vi "Command (read & write) - PR.vi"(7 "timeout ms (100)":i32=100, 8 "error in (no error)":errorcluster, 9 "Protocol Setting":i32, 10 "IP":string, 11 "connection ID in":refnum<k16>) -> (0 "error out":errorcluster, 2 "Protocol Setting":i32, 3 "connection ID out":refnum<k16>)   [LabVIEW 2016, in "SMD-7615.lvlib" / "eSCL.lvlib"]
doc: "PR - Protocol\nSets or requests the serial communication protocol settings. Sets or requests the serial communication protocol\nsettings. There are a number of settings that can be turned on or off in the PR command. Each setting is\nassigned a bit in a 9 - bit binary word. The parameter of the PR command is the decimal equivalent of this word. If you send the PR command without a parameter the drive will respond with the decimal equivalent of the word as well. The different protocol settings and their bit assignments are shown below."
uses:
  eSCL.lvlib
  I32 Command and Param.ctl
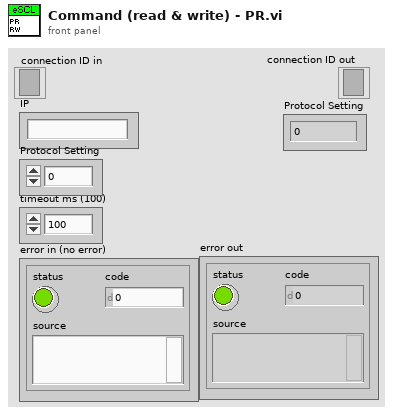
[diagram p1: front panel]
types:
  T1 = typedef "SMD-7615.lvlib/eSCL.lvlib/I32 Command and Param.ctl" = cluster{"Command":string, "I32 Parameler":i32, "I32 Parameler Default":i32, "I32 Parameler Coerece Upper":i32, "I32 Parameler Coerece Lower":i32}
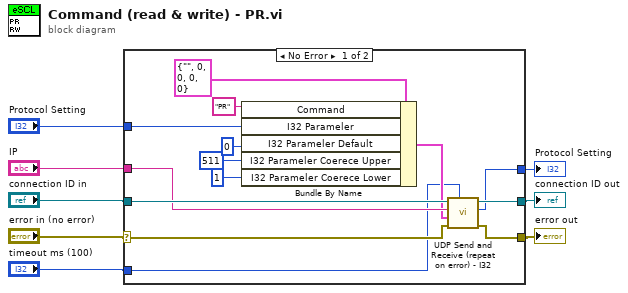
[diagram p0: block diagram]
diagram:
  n1 = case shown="No Error" "error in (no error)" {
    selector: "error in (no error)" -> [w16 w23]
    tunnel: "connection ID in" -> [w19 w24]
    tunnel: [w14 w24] -> w2
    tunnel: [w13 w23] -> w1
    tunnel: "IP" -> [w18 _]
    tunnel: "timeout ms (100)" -> [w15 _]
    tunnel: [w12 _] -> w8
    tunnel: "Protocol Setting" -> [w9 _]
    frame No Error {
      n2 = Bundle By Name(cluster=T1 {"Command"="", "I32 Parameler"=0, "I32 Parameler Default"=0, "I32 Parameler Coerece Upper"=0, "I32 Parameler Coerece Lower"=0} ("I32 Command & Param"), "Command"="PR", "I32 Parameler"=w9, "I32 Parameler Default"=0 ("DBL Parameler Default"), "I32 Parameler Coerece Upper"=511 ("DBL Parameler Coerece Upper"), "I32 Parameler Coerece Lower"=1 ("DBL Parameler Coerece Lower")) -> (w17:T1)
      n3 = call "UDP Send and Receive (repeat on error) - I32.vi"("timeout ms (100)"=w15, "error in (no error)"=w16, "I32 Command & Param"=w17, "IP"=w18, "connection ID in"=w19) -> ("error out"=w13:errorcluster, "I32 Param out"=w12:i32, "connection ID out"=w14:refnum<k16>)  [unwired: 4 in]
    }
    frame Error {
    }
  }
  "connection ID out" <- w2
  "error out" <- w1
  "Protocol Setting" <- w8
